vi "poly_caller_control_ref_from_name_multi.vi"(8 "error in":errorcluster caption="Error in (no error)", 10 "control names":string[](array[string])) -> (0 "error out":errorcluster, 2 "control refs":refnum<vi>[](array[refnum]), 4 "found?":bool[](array[boolean]))   [LabVIEW 2015]
uses:
  poly_control_ref_from_name_multi.vi
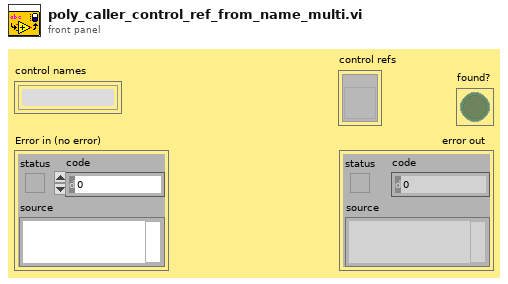
[diagram p1: front panel]
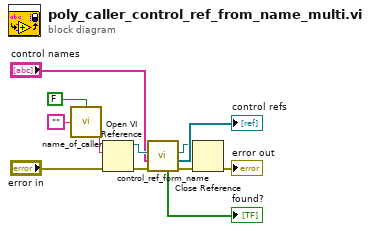
[diagram p0: block diagram]
diagram:
  n1 = call "name_of_caller.vi"("is in inlined vi? (F)"=FALSE, "name of caller in"="") -> ("name of caller out"=w10:string)  [unwired: 2 in]
  n2 = Open VI Reference(vi path=w10, error in (no error)="error in") -> (vi reference=w8:refnum<vi>, error out=w4:errorcluster)  [unwired: 4 in]
  n3 = call-poly "control_ref_form_name.vi"("error in (no error)"=w4, "control names"="control names", "vi ref"=w8) -> ("error out"=w2:errorcluster, "ctrl refs"=→"control refs":refnum<vi>[], "vi ref dup"=w3:refnum<vi>, "found?"=→"found?":bool[])  [unwired: 5 in]
  n4 = Close Reference(reference=w3, error in (no error)=w2) -> (error out=→"error out":errorcluster)
